vi "standard engine version.vi"() -> (3 "Version":string="1.0.0.0")   [LabVIEW 2013, in "Standard Engine Configuration.lvclass"]
uses:
  Standard Engine Configuration.lvclass
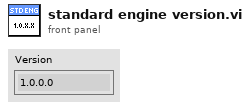
[diagram p1: front panel]
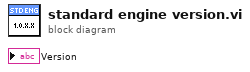
[diagram p0: block diagram]
diagram:
